vi "Configure Output.vi"(6 "Enable Transient Trigger Output (F: Disable)":bool, 8 "error in (no error)":errorcluster, 9 "Output Transient Mode (0: Fixed)":u16(ring) items=["Fixed", "Step", "List", "Arbitrary"], 10 "Output Priority Mode (0: Voltage)":u16(ring) items=["Voltage", "Current"], 11 "VISA resource name":refnum<visa-resource-name>) -> (0 "error out":errorcluster, 3 "VISA resource name out":refnum<visa-resource-name>)   [LabVIEW 2022 SP3, in "Agilent N6900 N7900 Series.lvlib"]
doc: "Configures the output of the power source. Note that since this VI sets the priority mode, it MUST be called before the Configure voltage/current VIs"
uses:
  Agilent N6900 N7900 Series.lvlib
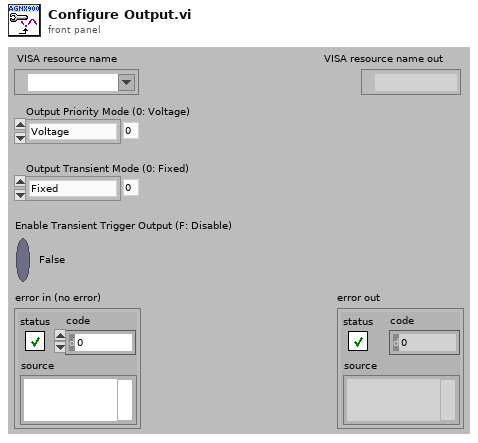
[diagram p1: front panel]
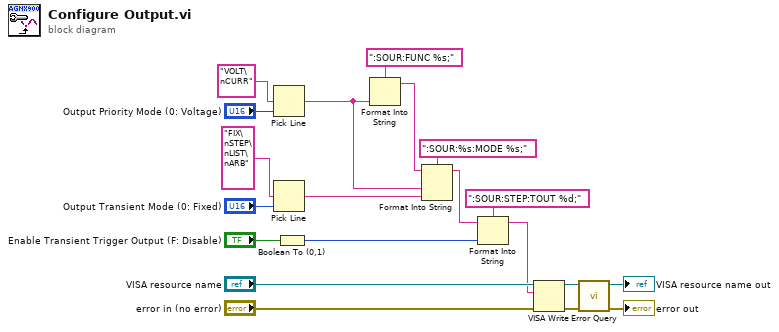
[diagram p0: block diagram]
diagram:
  n1 = Pick Line(multi-line string="VOLT\nCURR", line index="Output Priority Mode (0: Voltage)") -> (output string=w3:string)  [unwired: 1 in]
  n2 = Pick Line(multi-line string="FIX\nSTEP\nLIST\nARB", line index="Output Transient Mode (0: Fixed)") -> (output string=w6:string)  [unwired: 1 in]
  n3 = Boolean To (0,1)(Boolean="Enable Transient Trigger Output (F: Disable)") -> (0, 1=w13:i16)
  n4 = Format Into String(format string=":SOUR:FUNC %s;", w3) -> (resulting string=w4:string)  [unwired: 2 in, 1 out]
  n5 = Format Into String(format string=":SOUR:%s:MODE %s;", initial string=w4, w3, w6) -> (resulting string=w7:string)  [unwired: 1 in, 1 out]
  n6 = Format Into String(format string=":SOUR:STEP:TOUT %d;", initial string=w7, w13) -> (resulting string=w1:string)  [unwired: 1 in, 1 out]
  n7 = VISA Write(VISA resource name="VISA resource name", write buffer=w1, error in (no error)="error in (no error)") -> (VISA resource name out=w17:refnum<visa-resource-name>, error out=w18:errorcluster)  [unwired: 1 out]
  n8 = call "Error Query.vi"("error in (no error)"=w18, "VISA resource name"=w17) -> ("error out"=→"error out":errorcluster, "VISA resource name out"=→"VISA resource name out":refnum<visa-resource-name>)  [unwired: 6 in, 2 out]
